vi "Sorting_Process (SubVI).vi"(10 "Array in":string[](array[string]), 11 "Digital in":refnum<vi>) -> (1 "Boolean":bool, 2 "Array out":string[](array[string]), 3 "empty?":bool)   [LabVIEW 2019]
uses:
  ef11fdba-41bc-438e-bd4e-f5211ec413a3.vi
  <vilib>/numeric/Random Number (Range) DBL.vi
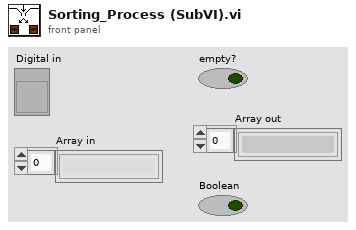
[diagram p1: front panel]
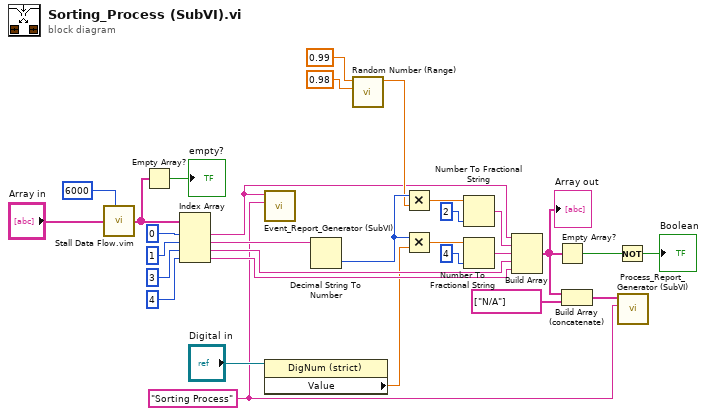
[diagram p0: block diagram]
diagram:
  w4 = "Sorting Process" ("Process Name")
  n1 = call "Stall Data Flow.vim"("value in"="Array in", "milliseconds to wait"=u32 6000) -> ("value out"=w25:string[])  [unwired: 1 out]
  n2 = Empty Array?(array=w25) -> (empty?=→"empty?":bool)
  n3 = Index Array(array=w25, index #1=0 ("index"), index #2=1 ("index"), index #3=3 ("index"), index #4=4 ("index")) -> (element #1=w5:string, element #2=w30:string, element #3=w27:string, element #4=w28:string)
  n4 = call "Event_Report_Generator (SubVI).vi"("Process Name"=w4, "Booking ID"=w5) -> ()  [unwired: 10 in]
  n5 = property class="DigNum (strict)"(reference="Digital in") -> ("Value"=w15:dbl)  [unwired: 1 in, 2 out]
  n6 = Decimal String To Number(string=w30) -> (number=w29:i32)  [unwired: 2 in, 1 out]
  n7 = call-poly <vilib>:"Random Number (Range).vi"("lower bound (0)"=0.98, "upper bound (100)"=0.99) -> ("number"=w18:dbl)  [unwired: 9 in]
  n8 = Multiply(x=w29, y=w18) -> (x*y=w11:dbl)
  n9 = Multiply(x=w29, y=w15) -> (x*y=w12:dbl)
  n10 = Number To Fractional String(number=w11, precision (6)=i16 2) -> (F-format string=w14:string)  [unwired: 2 in]
  n11 = Number To Fractional String(number=w12, precision (6)=i16 4) -> (F-format string=w13:string)  [unwired: 2 in]
  n12 = Build Array(w5, w14, w13, w27, w28) -> (w3:string[])
  "Array out" <- w3
  n13 = Empty Array?(array=w3) -> (empty?=w7:bool)
  n14 = Build Array (concatenate)(w3, string[] ["N/A"] ("array")) -> (w1:string[])
  n15 = Not(x=w7) -> (.not. x?=→"Boolean":bool)
  n16 = call "Process_Report_Generator (SubVI).vi"("Process Name"=w4, "Process Information"=w1) -> ()  [unwired: 10 in]
